vi "main.vi"() -> ()   [LabVIEW 2025]
panel:
  in  "对方端口":u16
  in  "对方IP":string
  out "服务器端口":u16
  out "服务器地址":u32
  out "UDP连接ID":refnum<k16>
  in  "客户端端口":u16
  out "接收区":string
  out "数据输出":string
  in  "发送":bool
  in  "发送区":string
  in  "发送新行":bool
  in  "打开连接":bool
  out "UDP状态":bool
  # "作为服务器发送数据"
  # "作为客户端读取数据"
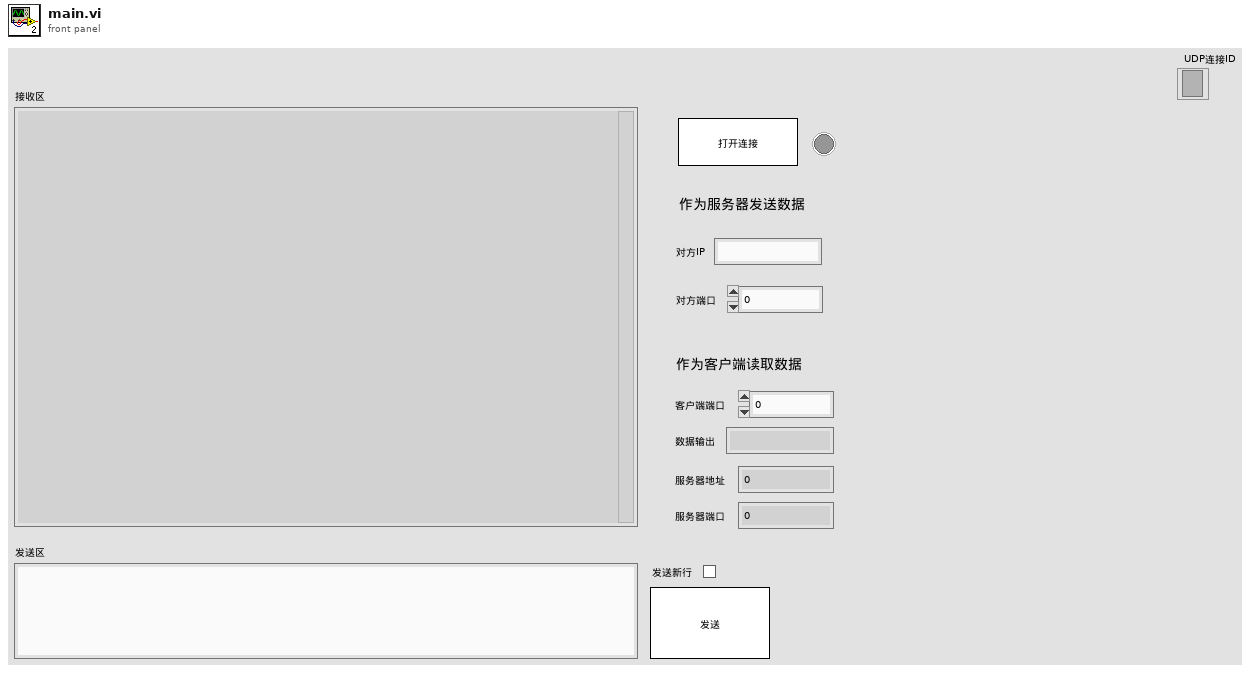
[diagram p1: front panel]
types:
  T1 = enum32{"invalid app kind", "Development System", "Run Time System", "Student Edition", "Embedded LabVIEW", "Evaluation", "Custom"}
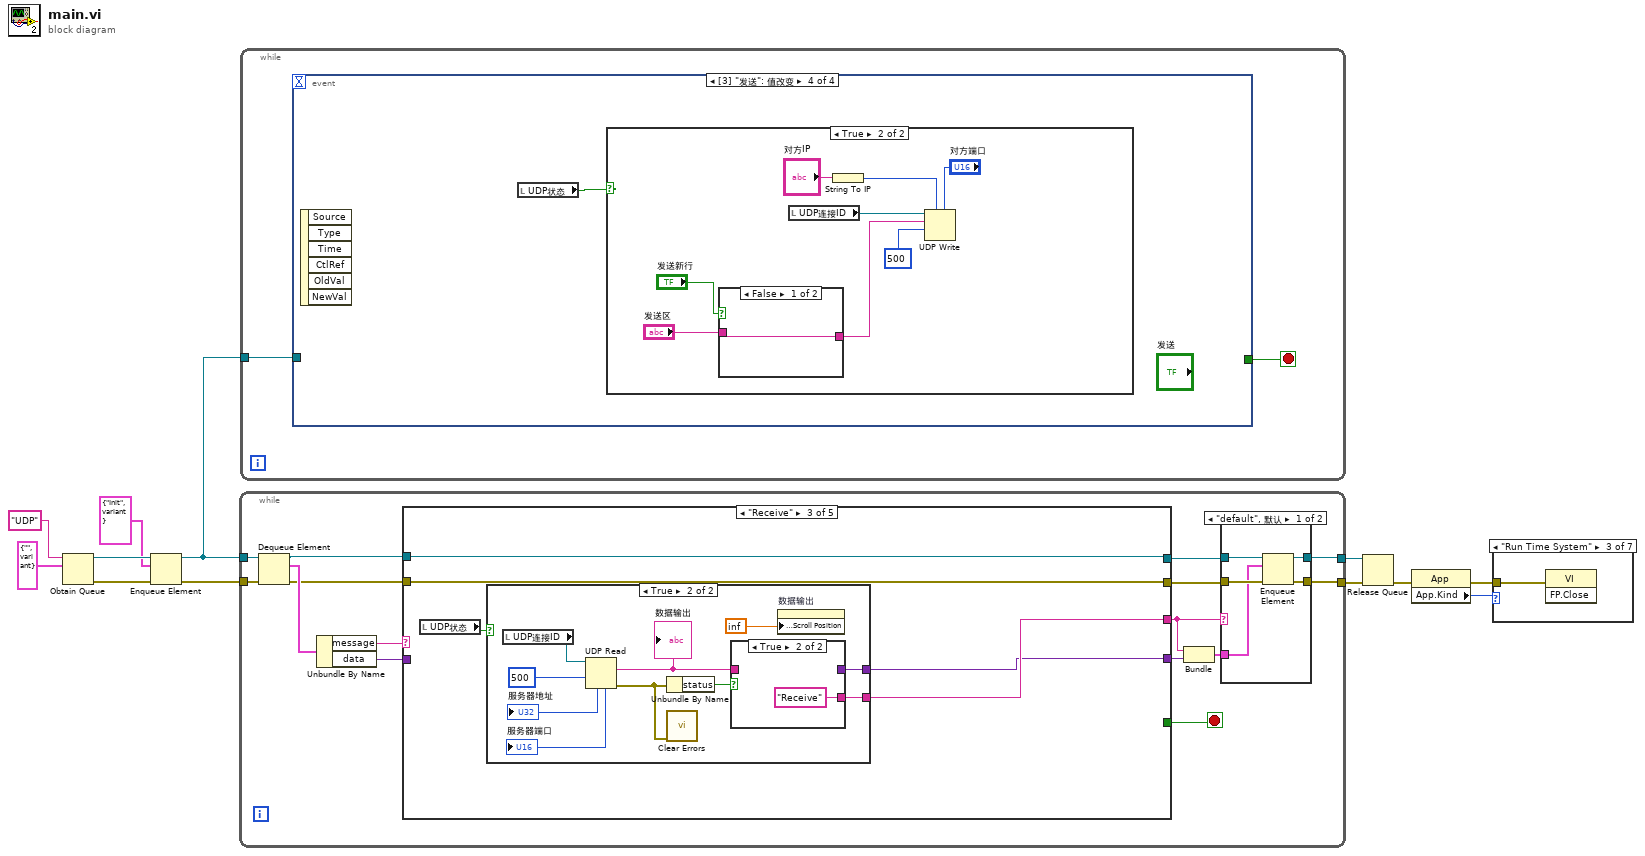
[diagram p0: block diagram]
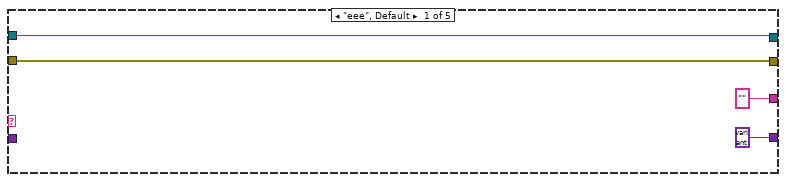
[diagram p9: hidden frame]
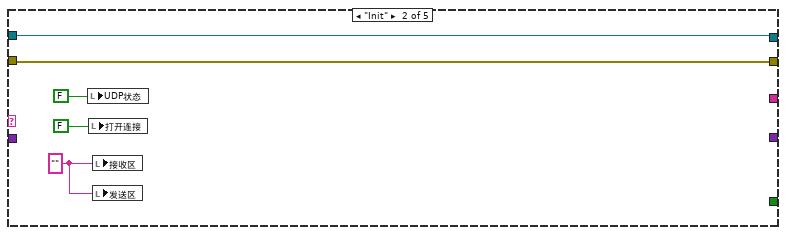
[diagram p10: hidden frame]
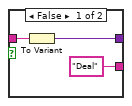
[diagram p12: hidden frame]
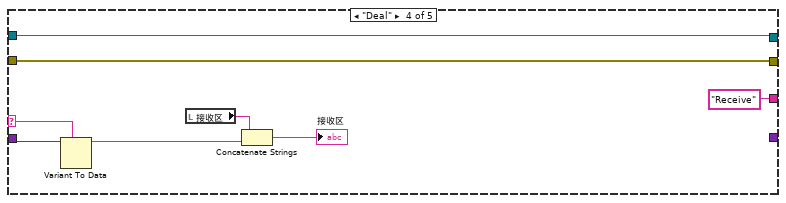
[diagram p13: hidden frame]
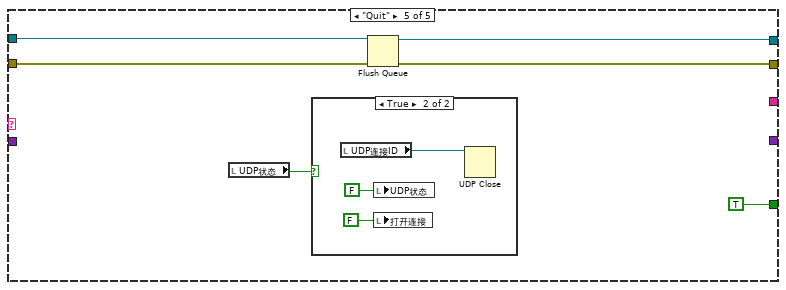
[diagram p14: hidden frame]
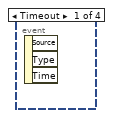
[diagram p16: hidden frame]
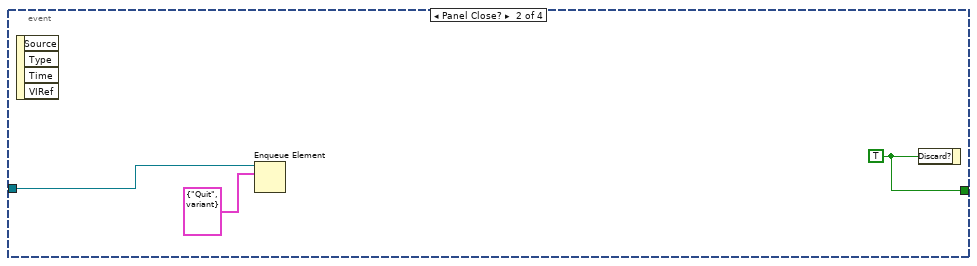
[diagram p17: hidden frame]
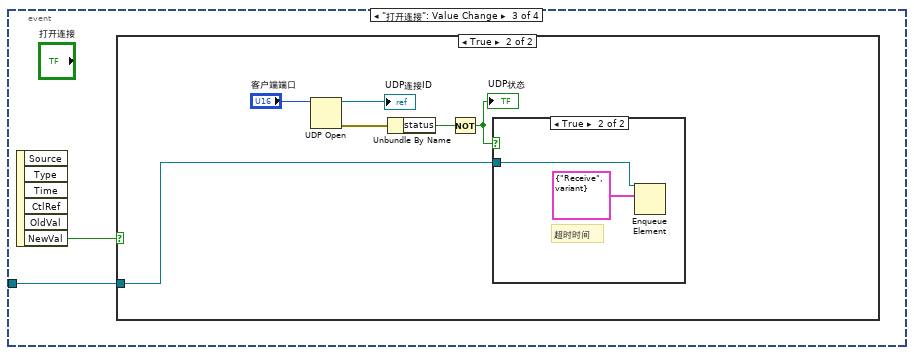
[diagram p18: hidden frame]
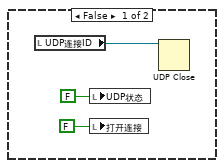
[diagram p19: hidden frame]
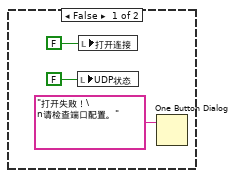
[diagram p20: hidden frame]
diagram:
  n1 = Obtain Queue(name (unnamed)="UDP" ("名称（未命名）"), element data type=cluster{"message":string, "data":variant} {"message"="", "data"=variant}) -> (queue out=w10:refnum<queue>, error out=w9:errorcluster)  [unwired: 3 in, 1 out]
  n2 = Enqueue Element(queue=w10, element=cluster{"message":string, "data":variant} {"message"="Init", "data"=variant} ("元素"), error in (no error)=w9) -> (queue out=w8:refnum<queue>, error out=w7:errorcluster)  [unwired: 1 in, 1 out]
  n3 = while {
    tunnel: w8 -> [w27]
    tunnel: w7 -> [w26]
    tunnel: [w17] -> w6
    tunnel: [w16] -> w5
    stop <- w15 stop-if-true
    n4 = Dequeue Element(queue=w27, error in (no error)=w26) -> (queue out=w23:refnum<queue>, element=w25:cluster{"message":string, "data":variant}, error out=w22:errorcluster)  [unwired: 1 in, 1 out]
    n5 = Unbundle By Name(w25) -> ("message"=w24:string, "data"=w19:variant)
    n6 = case shown="\"Receive\"" w24 {
      selector: w24 -> [_ _ _ w64 _]
      tunnel: [w38 w43 w48 w67 w75] -> w21
      tunnel: w23 -> [w38 w43 w48 w67 w74]
      tunnel: w22 -> [w37 w42 w46 w66 w73]
      tunnel: [w37 w42 w46 w66 w72] -> w20
      tunnel: ["" _ w45 "Receive" _] -> w13
      tunnel: w19 -> [_ _ _ w65 _]
      tunnel: [_ _ _ _ TRUE] -> w15
      tunnel: [variant _ w44 _ _] -> w14
      frame "eee", Default {
      }
      frame "Init" {
        w39 = "" ("UDP接收区")
        n7 = local write "UDP状态"(FALSE ("串口状态")) -> ()
        n8 = local write "打开连接"(FALSE ("串口开关")) -> ()
        n9 = local write "接收区"(w39) -> ()
        n10 = local write "发送区"(w39) -> ()
      }
      frame "Receive" {
        n11 = local read "UDP状态"() -> (w47:bool)
        n12 = case shown="True" w47 {
          tunnel: [_ w57] -> w45
          tunnel: [_ w56] -> w44
          frame False {
          }
          frame True {
            n13 = local read "UDP连接ID"() -> (w55:refnum<k16>)
            n14 = UDP Read(connection ID=w55, timeout ms (25000)=500 ("超时毫秒(25000)")) -> (data out=w51:string, error out=w50:errorcluster, 4:→"服务器端口":u16, 6:→"服务器地址":u32)  [unwired: 2 in, 1 out]
            "数据输出" <- w51
            n15 = Unbundle By Name(w50) -> ("status"=w58:bool)
            n16 = call <vilib>:"Clear Errors.vi"("error in (no error)"=w50) -> ()  [unwired: 5 in, 2 out]
            n17 = case shown="True" w58 {
              tunnel: ["Deal" "Receive"] -> w57
              tunnel: w51 -> [w60 _]
              tunnel: [w59 _] -> w56
              frame False {
                n18 = To Variant(anything=w60) -> (Variant=w59:variant)
              }
              frame True {
              }
            }
            n19 = property on="数据输出" class="Str"("Text.Scroll Position"=inf ("文本.滚动条位置")) -> ()  [unwired: 2 in, 2 out]
          }
        }
      }
      frame "Deal" {
        n20 = Variant To Data(type=w64, Variant=w65) -> (data=w63:string)  [unwired: 1 in, 1 out]
        n21 = local read "接收区"() -> (w69:string)
        n22 = Concatenate Strings(w69, w63) -> (→"接收区":string)
      }
      frame "Quit" {
        n23 = local read "UDP状态"() -> (w71:bool)
        n24 = case shown="True" w71 {
          frame False {
          }
          frame True {
            n25 = local read "UDP连接ID"() -> (w77:refnum<k16>)
            n26 = local write "UDP状态"(FALSE ("串口状态")) -> ()
            n27 = local write "打开连接"(FALSE ("串口开关")) -> ()
            n28 = UDP Close(connection ID=w77) -> ()  [unwired: 1 in, 2 out]
          }
        }
        n29 = Flush Queue(queue=w74, error in (no error)=w73) -> (queue out=w75:refnum<queue>, error out=w72:errorcluster)  [unwired: 1 out]
      }
    }
    n30 = Bundle(w13, "Variant"=w14) -> (w18:cluster{string, "Variant":variant})  [unwired: 1 in]
    n31 = case shown="\"default\", 默认" w13 {
      tunnel: w21 -> [w32 w34]
      tunnel: w20 -> [w31 w33]
      tunnel: w18 -> [w30 _]
      tunnel: [w29 w34] -> w17
      tunnel: [w28 w33] -> w16
      frame "default", Default {
        n32 = Enqueue Element(queue=w32, element=w30, error in (no error)=w31) -> (queue out=w29:refnum<queue>, error out=w28:errorcluster)  [unwired: 1 in, 1 out]
      }
      frame "" {
      }
    }
  }
  n33 = while {
    tunnel: w8 -> [w80]
    stop <- w81 stop-if-true
    n34 = event shown="[3] \"发送\": 值改变" {
      selector: _ -> [_ _ _ _]
      dyn-events: _ -> [_ _ _ _]
      timeout: _ -> [_ _ _ _]
      tunnel: [_ w84 _ _] -> w81
      tunnel: w80 -> [_ w83 w85 _]
      event Timeout {
        n35 = event-data() -> ()  [unwired: 1 in, 3 out]
      }
      event Panel Close? {
        w84 = TRUE ("放弃？")
        n36 = event-data() -> ()  [unwired: 1 in, 4 out]
        n37 = Enqueue Element(queue=w83, element=cluster{"message":string, "data":variant} {"message"="Quit", "data"=variant} ("元素")) -> ()  [unwired: 2 in, 3 out]
        n38 = event-data("Discard?"=w84) -> ()  [unwired: 1 in, 1 out]
      }
      event "打开连接": Value Change {
        n39 = event-data() -> ("NewVal"=w86:bool)  [unwired: 1 in, 5 out]
        n40 = case shown="True" w86 {
          tunnel: w85 -> [_ w93]
          frame False {
            n41 = local read "UDP连接ID"() -> (w87:refnum<k16>)
            n42 = local write "UDP状态"(FALSE ("串口状态")) -> ()
            n43 = local write "打开连接"(FALSE ("串口开关")) -> ()
            n44 = UDP Close(connection ID=w87) -> ()  [unwired: 1 in, 2 out]
          }
          frame True {
            n45 = UDP Open(11:"客户端端口") -> (port=→"UDP连接ID":refnum<k16>, 0:w90:errorcluster)  [unwired: 4 in, 1 out]
            n46 = Unbundle By Name(w90) -> ("status"=w94:bool)
            n47 = Not(x=w94) -> (.not. x?=w95:bool)
            "UDP状态" <- w95
            n48 = case shown="True" w95 {
              tunnel: w93 -> [_ w100]
              frame False {
                n49 = local write "UDP状态"(FALSE ("串口状态")) -> ()
                n50 = local write "打开连接"(FALSE ("串口开关")) -> ()
                n51 = One Button Dialog(message="打开失败！\n请检查端口配置。") -> ()  [unwired: 1 in, 1 out]
              }
              frame True {
                # "超时时间"
                n52 = Enqueue Element(queue=w100, element=cluster{"message":string, "data":variant} {"message"="Receive", "data"=variant} ("元素")) -> ()  [unwired: 2 in, 3 out]
              }
            }
          }
        }
      }
      event "发送": Value Change {
        n53 = event-data() -> ()  [unwired: 1 in, 6 out]
        n54 = local read "UDP状态"() -> (w101:bool)
        n55 = case shown="True" w101 {
          frame False {
            n56 = One Button Dialog(message="服务器未连接！") -> ()  [unwired: 1 in, 1 out]
          }
          frame True {
            n57 = case shown="False" "发送新行" {
              tunnel: "发送区" -> [w111 w114]
              tunnel: [w111 w112] -> w107
              frame False {
              }
              frame True {
                n58 = Concatenate Strings(w114, "\r\n" ("字符串")) -> (w112:string)
              }
            }
            n59 = local read "UDP连接ID"() -> (w108:refnum<k16>)
            n60 = String To IP(1:"对方IP") -> (0:w104:u32)
            n61 = UDP Write(address=w104, port or service name="对方端口", connection ID=w108, data in=w107, 9:500 ("超时毫秒(25000)")) -> ()  [unwired: 1 in, 2 out]
          }
        }
      }
    }
  }
  n62 = Release Queue(queue=w6, error in (no error)=w5) -> (error out=w4:errorcluster)  [unwired: 1 in, 2 out]
  n63 = property class="App"(error in=w4) -> (error out=w3:errorcluster, "App.Kind"=w1:T1)  [unwired: 1 in, 1 out]
  n64 = case shown="\"Run Time System\"" w1 {
    tunnel: w3 -> [_ _ w115 _ _ _ _]
    frame "invalid app kind", Default {
    }
    frame "Development System" {
    }
    frame "Run Time System" {
      n65 = invoke class="VI" method="FP.Close"(error in=w115) -> ()  [unwired: 2 in, 3 out]
    }
    frame "Student Edition" {
    }
    frame "Embedded LabVIEW" {
    }
    frame "Evaluation" {
    }
    frame "Custom" {
    }
  }
